vi "setpoint and rotate in steps.vi"(0 "axis 1: sp":dbl, 1 "final m/c temp setpoint":dbl, 5 "move axis 1":bool=TRUE, 7 "axis 2: sp":dbl, 9 "move axis 2":bool=TRUE, 11 "error in":errorcluster) -> (15 "error out":errorcluster)   [LabVIEW 2019]
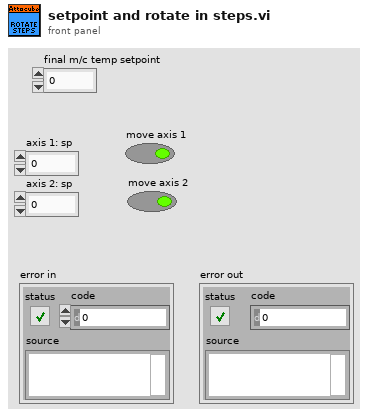
[diagram p1: front panel]
types:
  T1 = cluster{"axis 1: Current position (°)":dbl, "axis 2: Current position (°)":dbl, "axis 1: rot. count":dbl, "axis 2: rot. count":dbl, "axis 1: StepWidth":dbl, "axis 2: StepWidth":dbl, "axis 1: speed (°/s)":dbl, "axis 2: speed (°/s)":dbl, "axis 1: positioner status":cluster{"moving":bool, "stop detected":bool, "sensor error":bool, "sensor disconnected":bool}, "axis 2: positioner status":cluster{"moving":bool, "stop detected":bool, "sensor error":bool, "sensor disconnected":bool}}
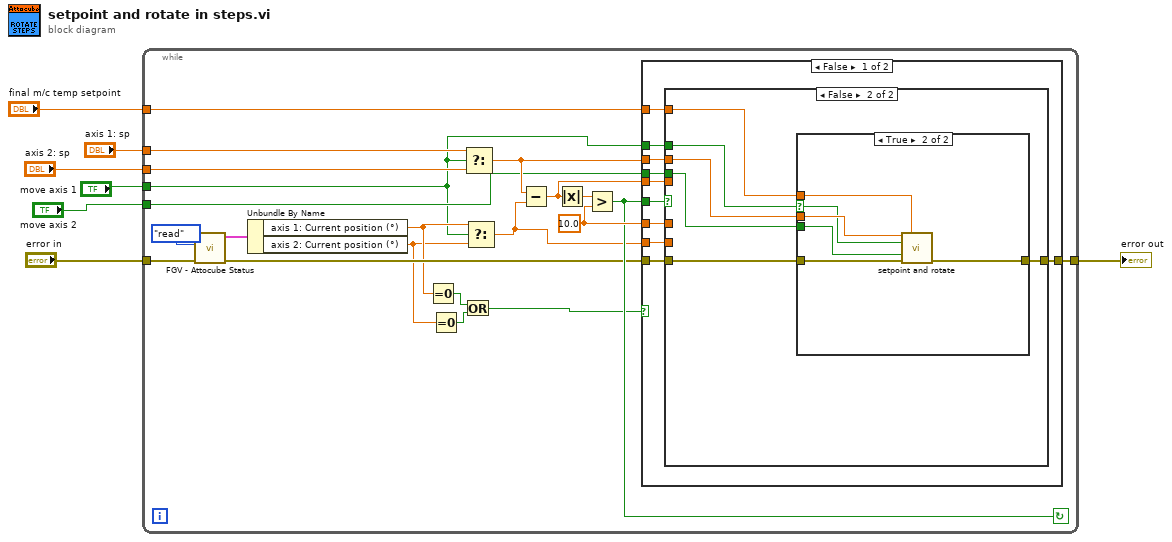
[diagram p0: block diagram]
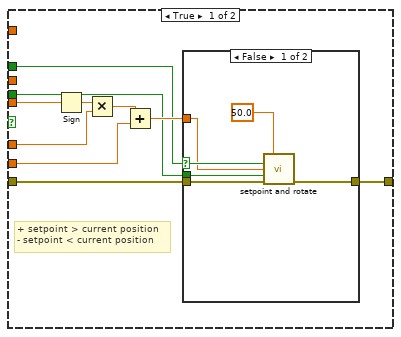
[diagram p2: hidden frame]
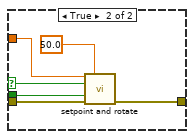
[diagram p3: hidden frame]
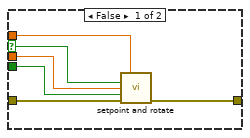
[diagram p4: hidden frame]
diagram:
  n1 = while {
    tunnel: "axis 1: sp" -> [w22]
    tunnel: "move axis 1" -> [w9]
    tunnel: "move axis 2" -> [w14]
    tunnel: "axis 2: sp" -> [w21]
    tunnel: "final m/c temp setpoint" -> [w20]
    tunnel: "error in" -> [w19]
    tunnel: [w17] -> w1
    stop <- w24 continue-if-true
    w25 = 10.0 ("y")
    n2 = call "FGV - Attocube Status.vi"("error in"=w19, "Function"=enum16{"write", "read"}."read") -> ("error out"=w18:errorcluster, "Status OUT"=w28:T1)  [unwired: 4 in]
    n3 = Unbundle By Name(w28) -> ("axis 1: Current position (°)"=w13:dbl, "axis 2: Current position (°)"=w12:dbl)
    n4 = Equal To 0?(x=w13) -> (x = 0?=w10:bool)
    n5 = Equal To 0?(x=w12) -> (x = 0?=w11:bool)
    n6 = Or(x=w10, y=w11) -> (x .or. y?=w8:bool)
    n7 = Select(t=w22, s=w9, f=w21) -> (s? t:f=w15:dbl)
    n8 = Select(t=w13, s=w9, f=w12) -> (s? t:f=w23:dbl)
    n9 = Subtract(x=w15, y=w23) -> (x-y=w26:dbl)
    n10 = Absolute Value(x=w26) -> (abs(x)=w27:dbl)
    n11 = Greater?(x=w27, y=w25) -> (0:w24:bool)
    n12 = case shown="False" w8 {
      tunnel: w26 -> [w38 _]
      tunnel: w25 -> [w37 _]
      tunnel: w24 -> [w36 _]
      tunnel: w23 -> [w35 _]
      tunnel: w20 -> [w34 _]
      tunnel: w18 -> [w33 w79]
      tunnel: [w32 w79] -> w17
      tunnel: w15 -> [w31 _]
      tunnel: w14 -> [w30 _]
      tunnel: w9 -> [w29 _]
      frame False {
        n13 = case shown="False" w36 {
          tunnel: w31 -> [_ w66]
          tunnel: w38 -> [w48 _]
          tunnel: w37 -> [w43 _]
          tunnel: w35 -> [w45 _]
          tunnel: w29 -> [w39 w65]
          tunnel: w30 -> [w42 w64]
          tunnel: w34 -> [_ w63]
          tunnel: w33 -> [w41 w62]
          tunnel: [w40 w61] -> w32
          frame True {
            # "+ setpoint > current position\n- setpoint < current position"
            n14 = Sign(1:w48) -> (0:w47:dbl)
            n15 = Multiply(x=w47, y=w43) -> (x*y=w46:dbl)
            n16 = Add(x=w46, y=w45) -> (x+y=w44:dbl)
            n17 = case shown="False" w39 {
              selector: w39 -> [w54 w59]
              tunnel: w44 -> [w49 w60]
              tunnel: w42 -> [w53 w58]
              tunnel: w41 -> [w52 w57]
              tunnel: [w51 w56] -> w40
              frame False {
                n18 = call "setpoint and rotate.vi"("m/c temp setpoint"=50.0, "move axis 1"=w54, "axis 2: sp position °"=w49, "move axis 2"=w53, "error in"=w52) -> ("error out"=w51:errorcluster)  [unwired: 9 in, 1 out]
              }
              frame True {
                n19 = call "setpoint and rotate.vi"("axis 1: sp position °"=w60, "m/c temp setpoint"=50.0, "move axis 1"=w59, "move axis 2"=w58, "error in"=w57) -> ("error out"=w56:errorcluster)  [unwired: 9 in, 1 out]
              }
            }
          }
          frame False {
            n20 = case shown="True" w65 {
              selector: w65 -> [w71 w77]
              tunnel: w66 -> [w72 w78]
              tunnel: w64 -> [w70 w76]
              tunnel: w63 -> [w69 w73]
              tunnel: w62 -> [w68 w75]
              tunnel: [w67 w74] -> w61
              frame False {
                n21 = call "setpoint and rotate.vi"("m/c temp setpoint"=w69, "move axis 1"=w71, "axis 2: sp position °"=w72, "move axis 2"=w70, "error in"=w68) -> ("error out"=w67:errorcluster)  [unwired: 9 in, 1 out]
              }
              frame True {
                n22 = call "setpoint and rotate.vi"("axis 1: sp position °"=w78, "m/c temp setpoint"=w73, "move axis 1"=w77, "move axis 2"=w76, "error in"=w75) -> ("error out"=w74:errorcluster)  [unwired: 9 in, 1 out]
              }
            }
          }
        }
      }
      frame True {
        # "if read 0 for either angle do nothing and try again"
      }
    }
  }
  "error out" <- w1
